vi "EnumerateDataTypes.vi"(8 "error in (no error)":errorcluster) -> (0 "error out":errorcluster, 3 "Data Types":string[](array[string]))   [LabVIEW 2017, in "WebServiceImporter.lvlib" / "ProxyDll Generator.lvlib"]
uses:
  <vilib>/Platform/WebService/ProxyDll Generator/ProxyDll Generator.lvlib
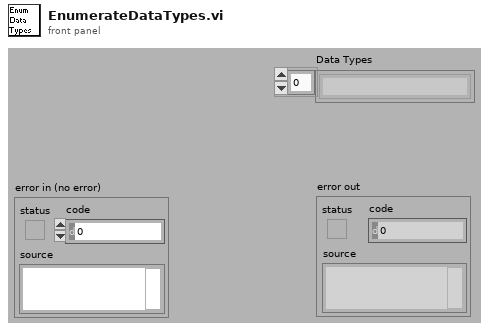
[diagram p1: front panel]
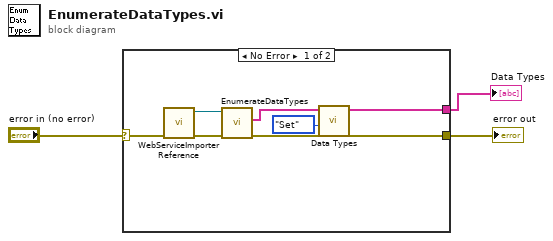
[diagram p0: block diagram]
diagram:
  n1 = case shown="No Error" "error in (no error)" {
    selector: "error in (no error)" -> [w9 w10]
    tunnel: [w7 w10] -> w2
    tunnel: [w4 _] -> w1
    frame No Error {
      n2 = call <vilib>:"WebServiceImporter Reference.vi"() -> ("Web Service Importer out"=w8:refnum<k24>)  [unwired: 10 in, 1 out]
      n3 = call <vilib>:"EnumerateDataTypes.vi"("error in (no error)"=w9, "Web Service Importer in"=w8) -> ("error out"=w7:errorcluster, "Data Types"=w5:string[])  [unwired: 7 in, 1 out]
      n4 = call <vilib>:"Data Types.vi"("Operation"=enum16{"Get", "Set"}."Set", "Data Types"=w5) -> ("Data Types (out)"=w4:string[])  [unwired: 8 in, 1 out]
    }
    frame Error {
    }
  }
  "Data Types" <- w1
  "error out" <- w2
